vi "Update SCADA PSP vars from OPCUA.vi"(8 "error in (no error)":errorcluster, 9 "CVT Array":T1[](array[typedef]), 10 "Variables":refnum<k21>[](array[refnum]), 11 "reference":refnum<k24>) -> (0 "error Out":errorcluster)   [LabVIEW 2019]
uses:
  <vilib>/NI/Current Value Table/Type Defs/Single Tag.ctl
  <vilib>/NI/Current Value Table/Type Defs/Data Types.ctl
  F:/src/HUTCDLSVN/Machine/CDL0100/TagEngine/LVOPCUA.NET/LVOPC.NETInterface/bin/Release/LVOPC.NETInterface.dll
  LVOPCUA.NET/LVOPC.NETInterface/bin/Release/LVOPC.NETInterface.dll
  <vilib>/NI/Current Value Table/Current Value Table.lvlib
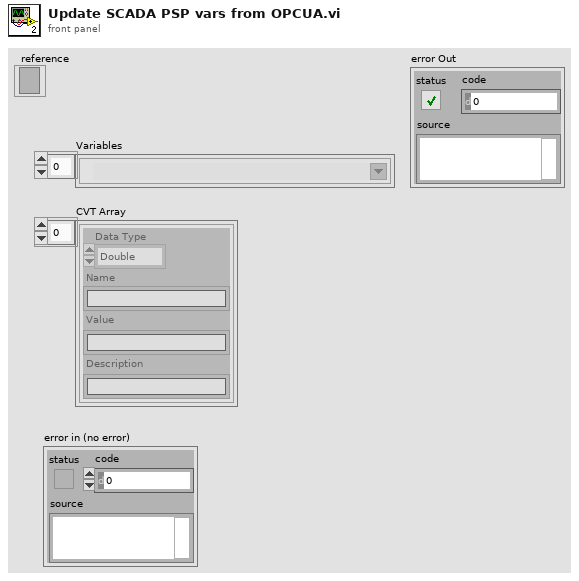
[diagram p1: front panel]
types:
  T1 = typedef "Current Value Table.lvlib/Single Tag.ctl" = cluster{"Data Type":T2, "Name":string, "Value":string, "Description":string}
  T2 = typedef "Current Value Table.lvlib/Data Types.ctl" = enum16{"Double", "Single", "I64", "I32", "I16", "I8", "U64", "U32", "U16", "U8", "String", "Boolean", "Array of U8", "Array of U16", "Array of U32", "Array of U64", "Array of I64", "Array of I32", "Array of I16", "Array of I8", "Array of Double", "Array of Single", "Array of Boolean", "Array of String"}
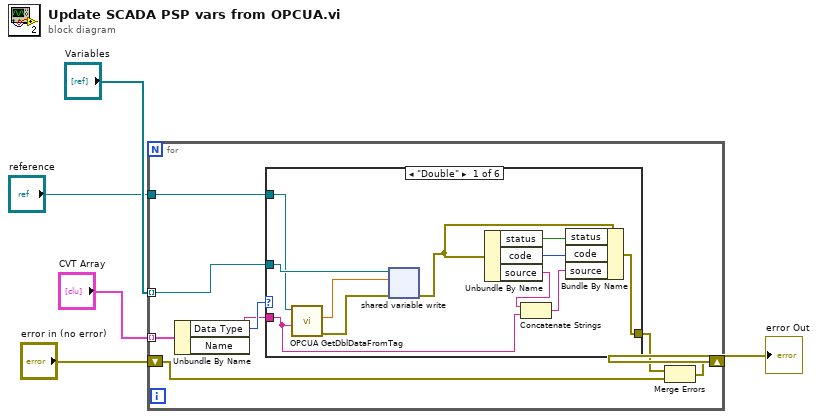
[diagram p0: block diagram]
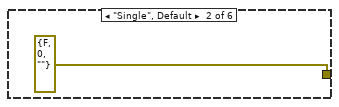
[diagram p2: hidden frame]
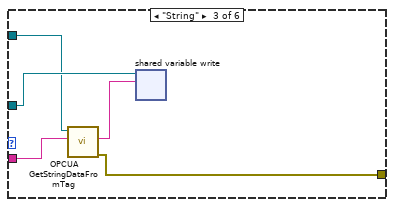
[diagram p3: hidden frame]
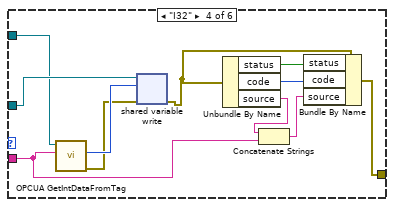
[diagram p4: hidden frame]
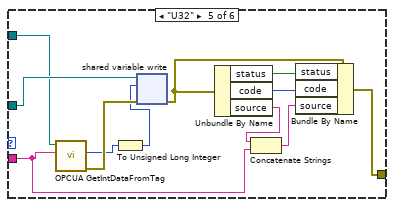
[diagram p5: hidden frame]
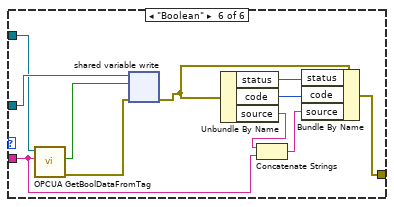
[diagram p6: hidden frame]
diagram:
  n1 = for {
    tunnel: "Variables" -> [w10] mode=indexing
    tunnel: "CVT Array" -> [w13] mode=indexing
    shift-right: [w7] -> w2
    shift-left: "error in (no error)" -> [w8]
    tunnel: "reference" -> [w6]
    n2 = Unbundle By Name(w13) -> ("Data Type"=w12:T2, "Name"=w11:string)
    n3 = case shown="\"Double\"" w12 {
      tunnel: w11 -> [w14 _ w30 w31 w47 w54]
      tunnel: w10 -> [w24 _ w29 w41 w53 w64]
      tunnel: [w15 errorcluster {"status"=FALSE, "code"=0, "source"=""} ("error IO") w26 w32 w45 w55] -> w9
      tunnel: w6 -> [w21 _ w27 w39 w52 w63]
      frame "Double" {
        n4 = call "OPCUA GetDblDataFromTag.vi"("tag"=w14, "reference"=w21) -> ("error out"=w22:errorcluster, "value"=w23:dbl)  [unwired: 7 in, 1 out]
        n5 = shared-variable-write(w24, w22, w23) -> (w16:errorcluster)  [unwired: 1 out]
        n6 = Unbundle By Name(w16) -> ("status"=w19:bool, "code"=w18:i32, "source"=w20:string)
        n7 = Concatenate Strings(w20, w14) -> (w17:string)
        n8 = Bundle By Name(cluster=w16, "status"=w19, "code"=w18, "source"=w17) -> (w15:errorcluster)
      }
      frame "Single", Default {
      }
      frame "String" {
        n9 = call "OPCUA GetStringDataFromTag.vi"("tag"=w30, "reference"=w27) -> ("error out"=w26:errorcluster, "value"=w28:string)  [unwired: 7 in, 1 out]
        n10 = shared-variable-write(w29, w28) -> ()  [unwired: 1 in, 2 out]
      }
      frame "I32" {
        n11 = call "OPCUA GetIntDataFromTag.vi"("tag"=w31, "reference"=w39) -> ("error out"=w38:errorcluster, "value"=w40:i32)  [unwired: 7 in, 1 out]
        n12 = shared-variable-write(w41, w38, w40) -> (w33:errorcluster)  [unwired: 1 out]
        n13 = Unbundle By Name(w33) -> ("status"=w36:bool, "code"=w35:i32, "source"=w37:string)
        n14 = Concatenate Strings(w37, w31) -> (w34:string)
        n15 = Bundle By Name(cluster=w33, "status"=w36, "code"=w35, "source"=w34) -> (w32:errorcluster)
      }
      frame "U32" {
        n16 = call "OPCUA GetIntDataFromTag.vi"("tag"=w47, "reference"=w52) -> ("error out"=w51:errorcluster, "value"=w50:i32)  [unwired: 7 in, 1 out]
        n17 = To Unsigned Long Integer(number=w50) -> (unsigned 32bit integer=w49:u32)
        n18 = shared-variable-write(w53, w51, w49) -> (w46:errorcluster)  [unwired: 1 out]
        n19 = Unbundle By Name(w46) -> ("status"=w44:bool, "code"=w43:i32, "source"=w48:string)
        n20 = Concatenate Strings(w48, w47) -> (w42:string)
        n21 = Bundle By Name(cluster=w46, "status"=w44, "code"=w43, "source"=w42) -> (w45:errorcluster)
      }
      frame "Boolean" {
        n22 = call "OPCUA GetBoolDataFromTag.vi"("tag"=w54, "reference"=w63) -> ("error out"=w61:errorcluster, "Value"=w62:bool)  [unwired: 7 in, 1 out]
        n23 = shared-variable-write(w64, w61, w62) -> (w56:errorcluster)  [unwired: 1 out]
        n24 = Unbundle By Name(w56) -> ("status"=w59:bool, "code"=w58:i32, "source"=w60:string)
        n25 = Concatenate Strings(w60, w54) -> (w57:string)
        n26 = Bundle By Name(cluster=w56, "status"=w59, "code"=w58, "source"=w57) -> (w55:errorcluster)
      }
    }
    n27 = Merge Errors(w9, w8) -> (w7:errorcluster)
  }
  "error Out" <- w2
